vi "Assert Check If Has course.vi"() -> ()   [LabVIEW 2015, in "Member_Actor.lvlib" / "TimeTable.lvclass"]
uses:
  TimeTable.lvclass
panel:
  out "Array":string[][](array[string])
  in  "CurWeek(0)":i32
  in  "SheetName(\"\")":string
  in  "Path":path
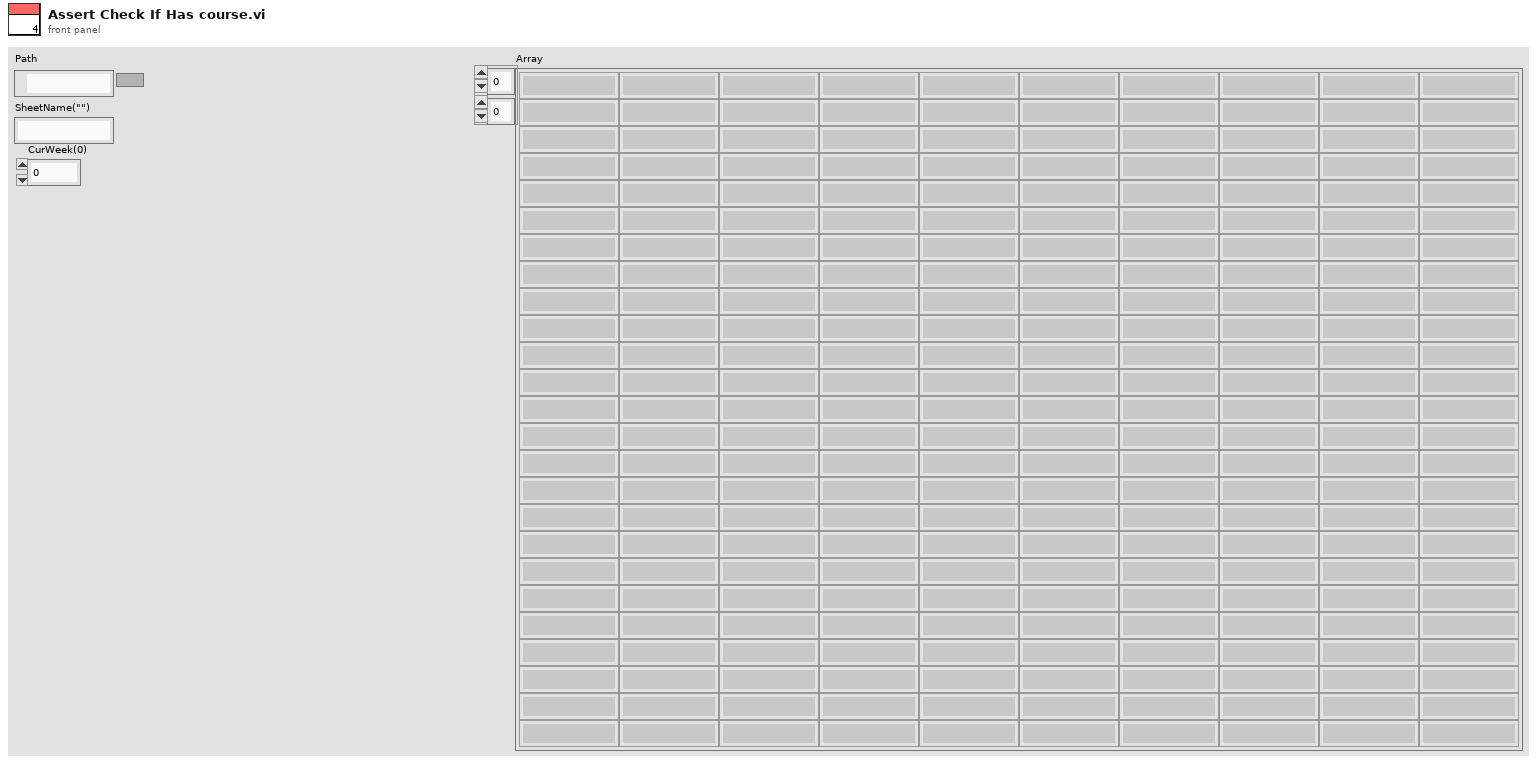
[diagram p1: front panel]
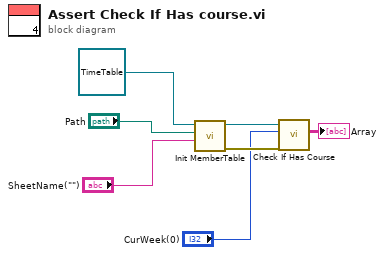
[diagram p0: block diagram]
diagram:
  n1 = call "Init MemberTable.vi"("SheetName(\"\")"="SheetName(\"\")", "Path"="Path", "TimeTable in"=refnum<class "TimeTable.lvclass"> refnum) -> ("error out"=w3:errorcluster, "TimeTable out"=w4:refnum<class "TimeTable.lvclass">)  [unwired: 7 in]
  n2 = call "Check If Has Course.vi"("error in (no error)"=w3, "CurWeek(0)"="CurWeek(0)", "TimeTable in"=w4) -> ("Array"=→"Array":string[][])  [unwired: 6 in, 2 out]
